vi "DownloadStatus..Callback.vi"(4 "User Parameter":variant, 5 "Event Data":cluster{"fileSize":i64, "status":u64}, 6 "Control Ref":refnum<k24>, 7 "Event Common Data":T1) -> ()   [LabVIEW 2019, in "LabSFTP.lvlib"]
uses:
  LabSFTP.lvlib
  C:/Users/1/Desktop/Pipeline leakage monitoring/V1.51-2020-8-10/References/LabSFTP.dll
  References/LabSFTP.dll
panel:
  # "Make Non Re-entrant"
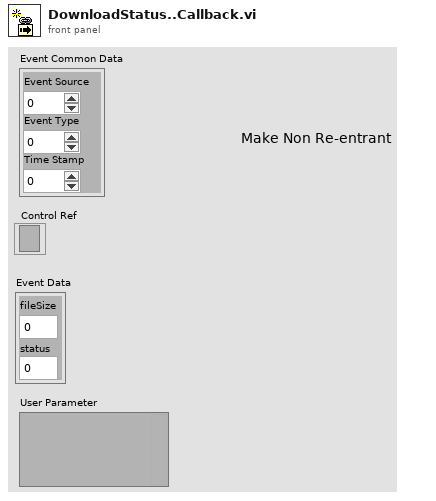
[diagram p1: front panel]
types:
  T1 = cluster{"Event Source":i32, "Event Type":u32, "Time Stamp":u32}
  T2 = typedef "LabSFTP.lvlib/Event Refs.ctl" = cluster{"UploadStatus":refnum<user-event>, "Stop":refnum<user-event>, "DownloadStatus":refnum<user-event>}
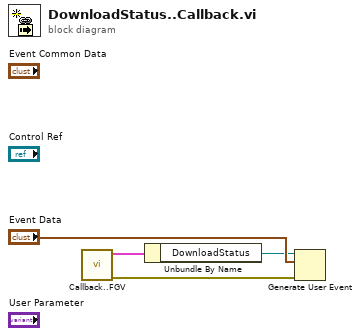
[diagram p0: block diagram]
diagram:
  n1 = call "Callback..FGV.vi"() -> ("error out"=w3:errorcluster, "Events"=w4:T2)  [unwired: 10 in]
  n2 = Unbundle By Name(w4) -> ("DownloadStatus"=w1:refnum<user-event>)
  n3 = Generate User Event(user event=w1, event data cluster="Event Data", error in=w3) -> ()  [unwired: 1 in, 2 out]
